vi "Reset.vi"(8 "error in (no error)":errorcluster, 9 "Timeout (5000 ms)":u32=5000, 10 "Reset Type (Warmstart)":u16(ring)=1 items=["Hotstart"=0, "Warmstart"=1, "Coldstart"=255], 11 "VISA resource name":refnum<visa-resource-name>) -> (0 "error out":errorcluster, 2 "Reset Successful":bool, 3 "VISA resource name out":refnum<visa-resource-name>)   [LabVIEW 2011, in "u-blox 5 Series.lvlib"]
doc: "Resets the instrument and waits until acknowledgment that the reset command has been received, or the timeout has been reached."
uses:
  u-blox 5 Series.lvlib
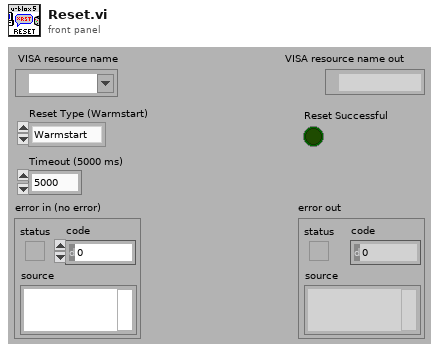
[diagram p1: front panel]
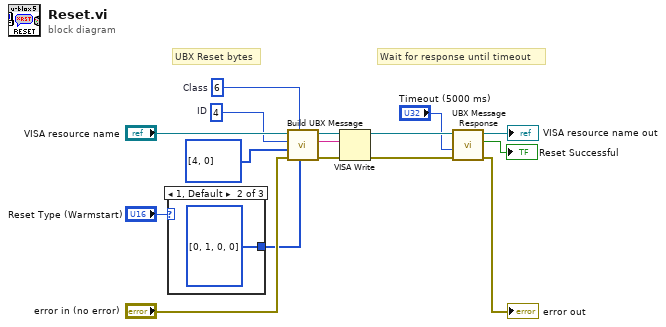
[diagram p0: block diagram]
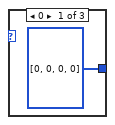
[diagram p2: hidden frame]
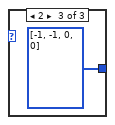
[diagram p3: hidden frame]
diagram:
  w1 = i8 4  # ID
  w11 = i8 6  # Class
  # "Wait for response until timeout"
  # "UBX Reset bytes"
  n1 = case shown="1, Default" "Reset Type (Warmstart)" {
    tunnel: [i8[] [0, 0, 0, 0] i8[] [0, 1, 0, 0] i8[] [-1, -1, 0, 0]] -> w4
    frame 0 {
    }
    frame 1, Default {
    }
    frame 2 {
    }
  }
  n2 = call "Build UBX Message.vi"("Payload"=w4, "Class"=w11, "error in"="error in (no error)", "Length"=i8[] [4, 0], "ID"=w1, "VISA resource name"="VISA resource name") -> ("error out"=w13:errorcluster, "UBX Message"=w12:string, "VISA resource name out"=w16:refnum<visa-resource-name>)  [unwired: 3 out]
  n3 = VISA Write(VISA resource name=w16, write buffer=w12, error in (no error)=w13) -> (VISA resource name out=w10:refnum<visa-resource-name>, error out=w9:errorcluster)  [unwired: 1 out]
  n4 = call "UBX Message Response.vi"("error in"=w9, "Timeout (1000 ms)"="Timeout (5000 ms)", "VISA resource name"=w10) -> ("error out"=→"error out":errorcluster, "Message Acknowledged"=→"Reset Successful":bool, "VISA resource name out"=→"VISA resource name out":refnum<visa-resource-name>)  [unwired: 1 in, 5 out]
